vi "MotorControl.vi"() -> ()   [LabVIEW 2022 SP3]
uses:
  <vilib>/Instr/_visa.llb/VISA Configure Serial Port (Instr).vi
panel:
  in  "clear":bool
  in  "Stop":bool
  out "Console":string
  in  "Cmds":enum32{"COM Port", "Run", "Advanced"}(tab)
  in  "Test":bool
  in  "VISA resource name":refnum<visa-resource-name>
  in  "Move":bool
  in  "desired steps":i16
  in  "Angle":i16(slide) scale=0.0..360.0
  in  "on":bool
  in  "off":bool
  in  "zero":bool
  in  "read":bool
  out "angle (deg)":i16
  in  "hit":bool
  in  "steps per degree":dbl=1.67
  in  "CntrlD":bool
  in  "Play Button":bool
  in  "String":string="turn(sm,100, True)\r\n"
  in  "Download":bool
  in  "CntrlC":bool
  # "sm.irq(flip)\nsm.active(1)\nturn(sm,100, True) # one Motor rotation CCW is 200 steps\nwhile running:\n    sleep(0.5)\n\nturn(sm,100, False)\nwhile running:\n    sleep(0.5)\n\nprint(\"done\")\nsm.active(0)\nsm.exec(\"set(pins,0)\")"
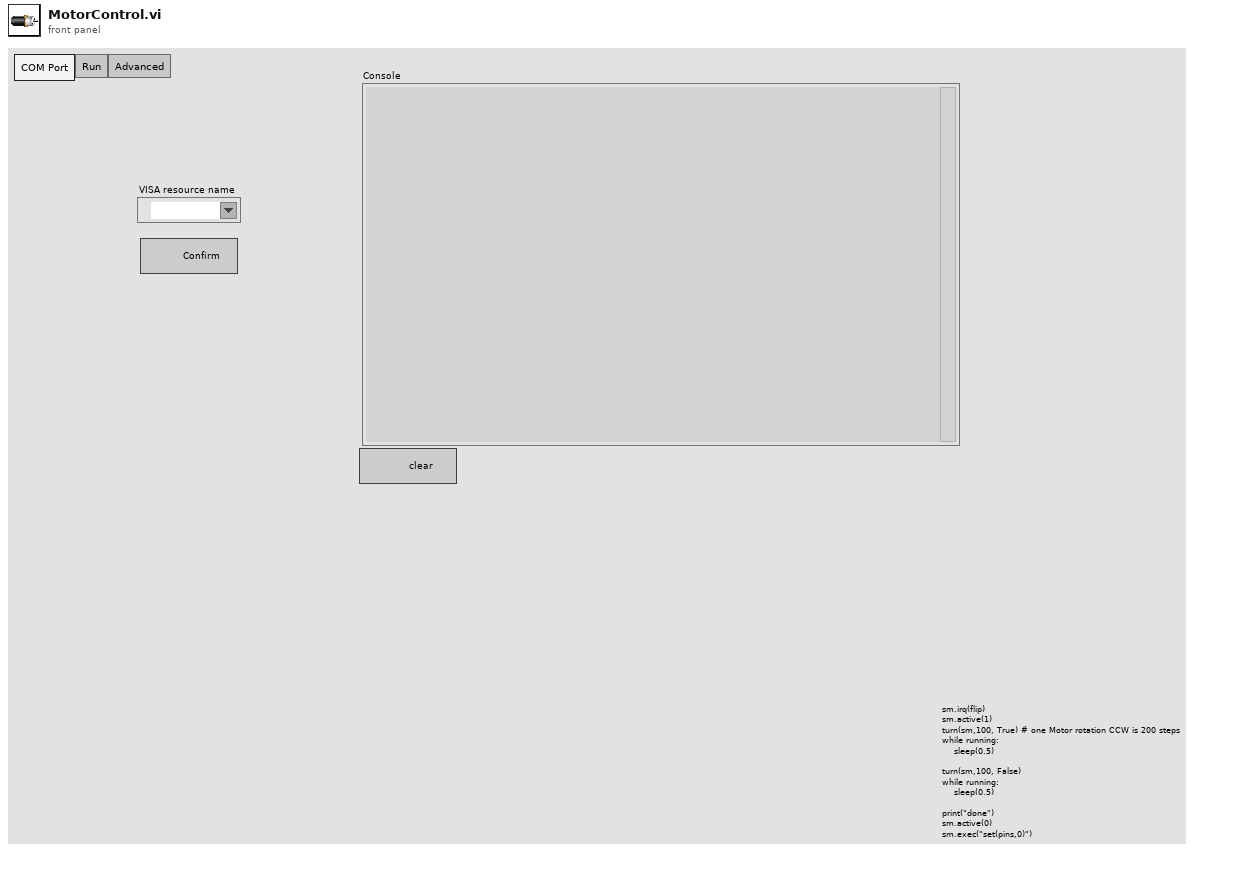
[diagram p1: front panel]
types:
  T1 = enum8{"Enabled", "Disabled", "Disabled and Grayed Out"}
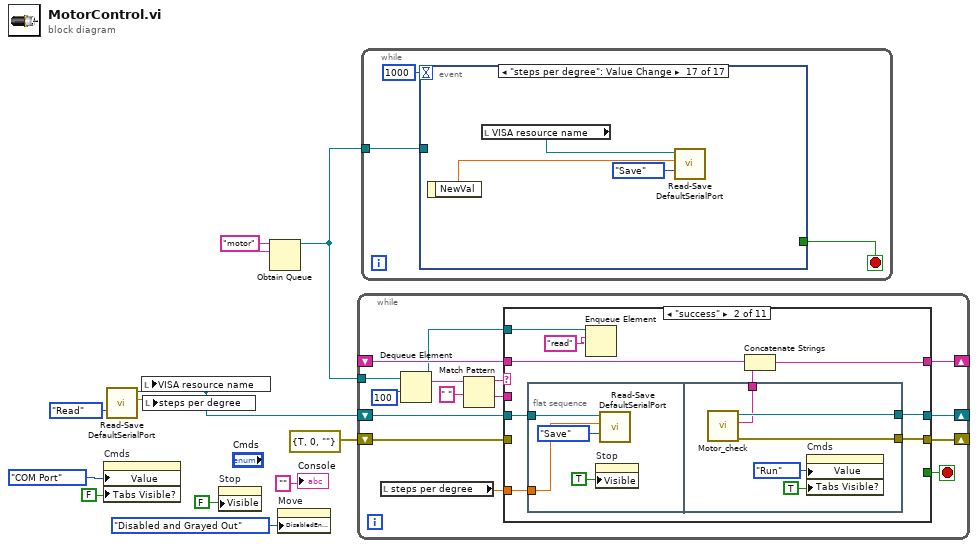
[diagram p0: block diagram]
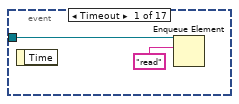
[diagram p2: hidden frame]
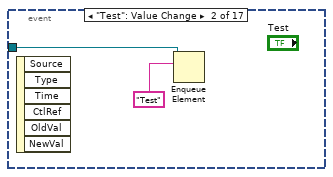
[diagram p3: hidden frame]
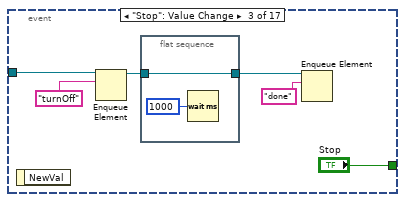
[diagram p4: hidden frame]
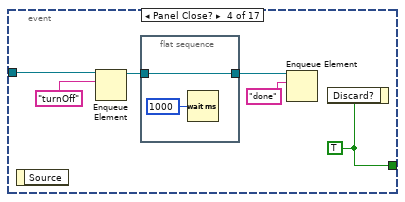
[diagram p5: hidden frame]
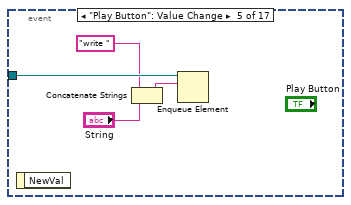
[diagram p6: hidden frame]
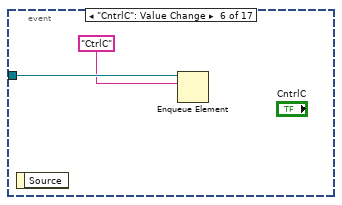
[diagram p7: hidden frame]
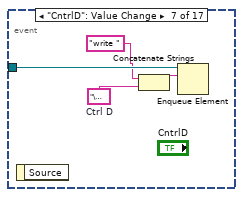
[diagram p8: hidden frame]
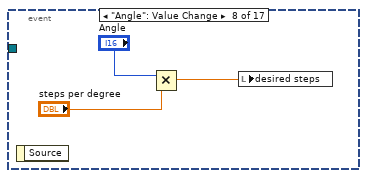
[diagram p9: hidden frame]
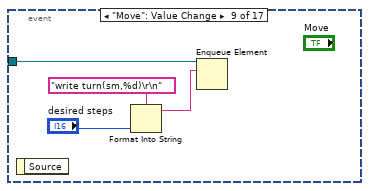
[diagram p10: hidden frame]
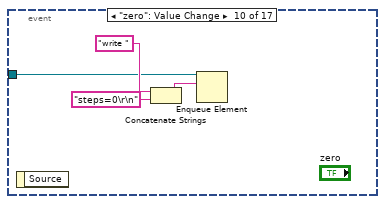
[diagram p11: hidden frame]
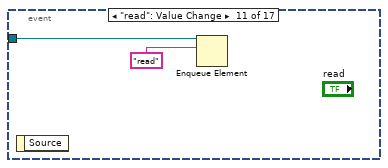
[diagram p12: hidden frame]
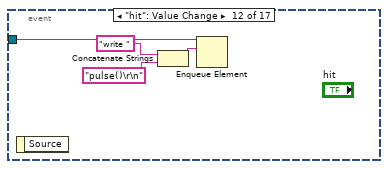
[diagram p13: hidden frame]
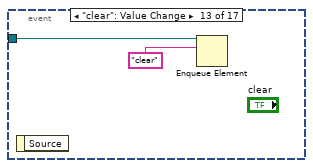
[diagram p14: hidden frame]
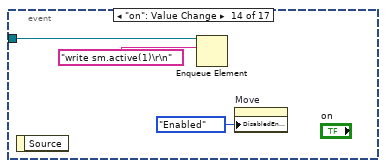
[diagram p15: hidden frame]
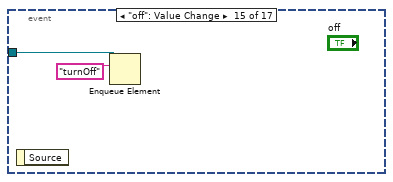
[diagram p16: hidden frame]
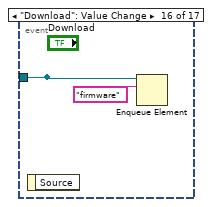
[diagram p17: hidden frame]
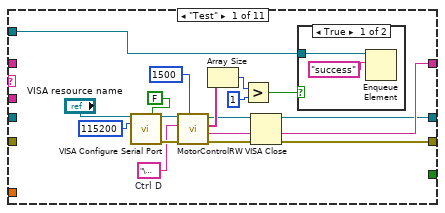
[diagram p18: hidden frame]
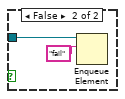
[diagram p19: hidden frame]
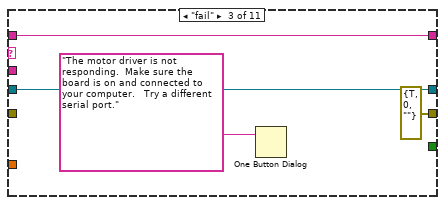
[diagram p20: hidden frame]
diagram:
  w5 = "motor" ("name (unnamed)")
  n1 = property on="Cmds" class="TabCtl (strict)"("Value"=enum32{"COM Port", "Run", "Advanced"}."COM Port" ("Cmds"), "Tabs Visible?"=FALSE) -> ()  [unwired: 2 in, 2 out]
  n2 = call "Read-Save DefaultSerialPort.vi"("Task"=enum16{"Save", "Read"}."Read") -> ("steps per degree out"=w1:dbl, "VISA out"=w4:refnum<visa-resource-name>)  [unwired: 8 in, 1 out]
  n3 = local write "VISA resource name"(w4) -> ()
  n4 = local write "steps per degree"(w1) -> ()
  n5 = property on="Stop" class="Bool"("Visible"=FALSE) -> ()  [unwired: 2 in, 2 out]
  n6 = Obtain Queue(name (unnamed)=w5, element data type=w5) -> (queue out=w3:refnum<queue>)  [unwired: 3 in, 2 out]
  n7 = property on="Move" class="Bool"("DisabledEnum"=T1."Disabled and Grayed Out" ("Disabled")) -> ()  [unwired: 2 in, 2 out]
  n8 = while {
    shift-right: [w24] -> _
    shift-left: _ -> [w25]
    tunnel: w3 -> [w22]
    shift-right: [w15] -> _
    shift-left: w4 -> [w26]
    shift-right: [w14] -> _
    shift-left: errorcluster {"status"=TRUE, "code"=0, "source"=""} ("error out") -> [w23]
    stop <- w16 stop-if-true
    n9 = local read "steps per degree"() -> (w12:dbl)
    n10 = Dequeue Element(queue=w22, timeout in ms (-1)=100) -> (queue out=w13:refnum<queue>, element=w20:string)  [unwired: 1 in, 2 out]
    n11 = Match Pattern(string=w20, regular expression=" ") -> (before substring=w19:string, after substring=w18:string)  [unwired: 1 in, 2 out]
    n12 = case shown="\"success\"" w19 {
      tunnel: w26 -> [_ w54 w66 w72 w79 w85 w94 w103 w112 w116 w127]
      tunnel: w25 -> [_ w50 w67 w68 w76 w83 w99 _ w113 w121 w126]
      tunnel: [w31 w49 w67 w69 w76 w83 w98 "" w113 w121 w125] -> w24
      tunnel: w23 -> [_ _ _ w73 w78 w84 w95 w102 w111 w117 w122]
      tunnel: w18 -> [_ _ _ _ w77 _ _ _ _ _ _]
      tunnel: [_ _ _ _ _ _ _ _ _ TRUE _] -> w16
      tunnel: [w28 w52 w66 w72 w75 w80 w97 w103 w106 w116 w124] -> w15
      tunnel: [w27 w53 errorcluster {"status"=TRUE, "code"=0, "source"=""} ("error out") w71 w74 w81 w96 w102 w105 w115 w123] -> w14
      tunnel: w13 -> [w29 w47 _ _ _ _ _ _ _ _ _]
      tunnel: w12 -> [_ w46 _ _ _ _ w86 _ _ _ _]
      frame "Test" {
        w34 = "\u0004"  # Ctrl D
        n13 = call-poly "VISA Configure Serial Port"("VISA resource name"="VISA resource name", "Enable Termination\nChar (T)"=FALSE ("Enable Termination\nChar (T)"), "baud rate (9600)"=u32 115200) -> ("VISA resource name out"=w38:refnum<visa-resource-name>, "error out"=w39:errorcluster)  [unwired: 11 in]
        n14 = call "MotorControlRW.vi"("timeout (msec)"=u32 1500 ("timeout"), "error in (no error)"=w39, "payload"=w34, "VISA in"=w38) -> ("error out"=w27:errorcluster, "reply"=w31:string, "rows"=w40:string[], "VISA Out"=w28:refnum<visa-resource-name>)  [unwired: 3 in, 1 out]
        n15 = Array Size(array=w40) -> (size(s)=w41:i32)
        n16 = Greater?(x=w41, y=1) -> (0:w30:bool)
        n17 = VISA Close(VISA resource name=w28, error in (no error)=w27) -> ()  [unwired: 1 out]
        n18 = case shown="True" w30 {
          tunnel: w29 -> [w42 w44]
          frame True {
            n19 = Enqueue Element(queue=w42, element="success") -> ()  [unwired: 2 in, 3 out]
          }
          frame False {
            n20 = Enqueue Element(queue=w44, element="fail") -> ()  [unwired: 2 in, 3 out]
          }
        }
      }
      frame "success" {
        n21 = flat-sequence {
          tunnel: w54 -> [w56]
          tunnel: w46 -> [w55]
          tunnel: [w63] -> w53
          tunnel: [w62] -> w52
          tunnel: [w59] -> w51
          frame #0 {
            n22 = property on="Stop" class="Bool"("Visible"=TRUE) -> ()  [unwired: 2 in, 2 out]
            n23 = call "Read-Save DefaultSerialPort.vi"("Task"=enum16{"Save", "Read"}."Save", "steps per degree"=w55, "VISA"=w56) -> ()  [unwired: 6 in, 3 out]
          }
          frame #1 {
            n24 = call "Motor_check.vi"() -> ("error out"=w63:errorcluster, "reply"=w59:string, "VISA Refnum out"=w62:refnum<visa-resource-name>)  [unwired: 8 in, 1 out]
            n25 = property on="Cmds" class="TabCtl (strict)"("Value"=enum32{"COM Port", "Run", "Advanced"}."Run" ("Cmds"), "Tabs Visible?"=TRUE) -> ()  [unwired: 2 in, 2 out]
          }
        }
        n26 = Enqueue Element(queue=w47, element="read") -> ()  [unwired: 2 in, 3 out]
        n27 = Concatenate Strings(w50, w51) -> (w49:string)
      }
      frame "fail" {
        n28 = One Button Dialog(message="The motor driver is not responding.  Make sure the board is on and connected to your computer.   Try a different serial port." ("regular expression")) -> ()  [unwired: 1 in, 1 out]
      }
      frame "firmware" {
        n29 = call "Motor_firmware.vi"("error in (no error)"=w73, "VISA Refnum in"=w72) -> ("error out"=w71:errorcluster, "reply"=w70:string)  [unwired: 8 in]
        n30 = Concatenate Strings(w68, w70) -> (w69:string)
      }
      frame "write" {
        n31 = VISA Write(VISA resource name=w79, write buffer=w77, error in (no error)=w78) -> (VISA resource name out=w75:refnum<visa-resource-name>, error out=w74:errorcluster)  [unwired: 1 out]
      }
      frame "CtrlC" {
        w82 = "\u0003"  # Ctrl C
        n32 = VISA Write(VISA resource name=w85, write buffer=w82, error in (no error)=w84) -> (VISA resource name out=w80:refnum<visa-resource-name>, error out=w81:errorcluster)  [unwired: 1 out]
      }
      frame "read" {
        w100 = "steps\r\n"  # steps?
        n33 = call "MotorControlRW.vi"("error in (no error)"=w95, "payload"=w100, "VISA in"=w94) -> ("error out"=w96:errorcluster, "reply"=w92:string, "rows"=w101:string[], "VISA Out"=w97:refnum<visa-resource-name>)  [unwired: 4 in, 1 out]
        n34 = Index Array(array=w101) -> (element #2=w90:string)  [unwired: 2 in, 1 out]
        n35 = Decimal String To Number(string=w90) -> (number=w89:i32)  [unwired: 2 in, 1 out]
        n36 = Match Pattern(string=w92, regular expression="steps") -> (before substring=w91:string)  [unwired: 1 in, 3 out]
        n37 = Divide(x=w89, y=w86) -> (x/y=w88:dbl)
        n38 = Round To Nearest(number=w88) -> (nearest integer value=→"angle (deg)":dbl)
        n39 = Concatenate Strings(w99, w91) -> (w98:string)
      }
      frame "clear" {
      }
      frame "turnOff" {
        w110 = "\u0003"  # Ctrl C
        n40 = VISA Write(VISA resource name=w112, write buffer=w110, error in (no error)=w111) -> (VISA resource name out=w109:refnum<visa-resource-name>, error out=w108:errorcluster)  [unwired: 1 out]
        n41 = VISA Write(VISA resource name=w109, write buffer="sm.active(0)\r\nsm.exec(\"set(pins,0)\")\r\n" ("element"), error in (no error)=w108) -> (VISA resource name out=w106:refnum<visa-resource-name>, error out=w105:errorcluster)  [unwired: 1 out]
        n42 = property on="Move" class="Bool"("DisabledEnum"=T1."Disabled and Grayed Out" ("Disabled")) -> ()  [unwired: 2 in, 2 out]
      }
      frame "done" {
        n43 = VISA Close(VISA resource name=w116, error in (no error)=w117) -> (error out=w115:errorcluster)
        n44 = property on="Cmds" class="TabCtl (strict)"("Value"=enum32{"COM Port", "Run", "Advanced"}."COM Port" ("Cmds"), "Tabs Visible?"=TRUE) -> ()  [unwired: 2 in, 2 out]
      }
      frame Default {
        n45 = case shown="No Error" w122 {
          selector: w122 -> [w128 w139]
          tunnel: w127 -> [w135 w140]
          tunnel: w126 -> [w133 w141]
          tunnel: [w132 w141] -> w125
          tunnel: [w130 w140] -> w124
          tunnel: [w129 w139] -> w123
          frame No Error {
            n46 = property class="Instr"(reference=w135, error in=w128) -> (reference out=w138:refnum<visa-resource-name>, error out=w136:errorcluster, "Serial Settings:Number of Bytes at Serial Port"=w137:u32)
            n47 = VISA Read(VISA resource name=w138, byte count=w137, error in (no error)=w136) -> (VISA resource name out=w130:refnum<visa-resource-name>, read buffer=w134:string, error out=w129:errorcluster)  [unwired: 1 out]
            n48 = Concatenate Strings(w133, w134) -> (w132:string)
            n49 = property on="Console" class="Str"("Value"=w132, "Text.Scroll Position"=u32 999999) -> ()  [unwired: 2 in, 2 out]
          }
          frame Error {
          }
        }
      }
    }
  }
  n50 = while {
    tunnel: w3 -> [w144]
    stop <- w143 stop-if-true
    n51 = event shown="[16] \"steps per degree\": Value Change" {
      selector: _ -> [_ _ _ _ _ _ _ _ _ _ _ _ _ _ _ _ _]
      dyn-events: _ -> [_ _ _ _ _ _ _ _ _ _ _ _ _ _ _ _ _]
      timeout: 1000 -> [_ _ _ _ _ _ _ _ _ _ _ _ _ _ _ _ _]
      tunnel: w144 -> [w146 w148 w152 w161 w168 w170 w174 _ w181 w183 w187 w191 w193 w196 w198 w200 _]
      tunnel: [_ _ "Stop" w157 _ _ _ _ _ _ _ _ _ _ _ _ _] -> w143
      tunnel: [_ _ _ _ _ _ _ _ _ _ _ _ _ _ _ w200 _] -> _
      event Timeout {
        n52 = event-data() -> ()  [unwired: 1 in, 1 out]
        n53 = Enqueue Element(queue=w146, element="read") -> ()  [unwired: 2 in, 3 out]
      }
      event "Test": Value Change {
        n54 = event-data() -> ()  [unwired: 1 in, 6 out]
        n55 = Enqueue Element(queue=w148, element="Test") -> ()  [unwired: 2 in, 3 out]
      }
      event "Stop": Value Change {
        n56 = event-data() -> ()  [unwired: 1 in, 1 out]
        n57 = Enqueue Element(queue=w152, element="turnOff") -> (queue out=w149:refnum<queue>)  [unwired: 2 in, 2 out]
        n58 = flat-sequence {
          tunnel: [w156] -> w150
          tunnel: w149 -> [w156]
          frame #0 {
            n59 = Wait (ms)(milliseconds to wait=u32 1000) -> ()  [unwired: 1 out]
          }
        }
        n60 = Enqueue Element(queue=w150, element="done") -> ()  [unwired: 2 in, 3 out]
      }
      event Panel Close? {
        w157 = TRUE
        n61 = event-data() -> ()  [unwired: 1 in, 1 out]
        n62 = Enqueue Element(queue=w161, element="turnOff") -> (queue out=w158:refnum<queue>)  [unwired: 2 in, 2 out]
        n63 = flat-sequence {
          tunnel: [w164] -> w159
          tunnel: w158 -> [w164]
          frame #0 {
            n64 = Wait (ms)(milliseconds to wait=u32 1000) -> ()  [unwired: 1 out]
          }
        }
        n65 = Enqueue Element(queue=w159, element="done") -> ()  [unwired: 2 in, 3 out]
        n66 = event-data("Discard?"=w157) -> ()  [unwired: 1 in, 1 out]
      }
      event "Play Button": Value Change {
        n67 = event-data() -> ()  [unwired: 1 in, 1 out]
        n68 = Concatenate Strings("write " ("element"), "String") -> (w165:string)
        n69 = Enqueue Element(queue=w168, element=w165) -> ()  [unwired: 2 in, 3 out]
      }
      event "CntrlC": Value Change {
        n70 = event-data() -> ()  [unwired: 1 in, 1 out]
        n71 = Enqueue Element(queue=w170, element="CtrlC") -> ()  [unwired: 2 in, 3 out]
      }
      event "CntrlD": Value Change {
        w172 = "\u0004"  # Ctrl D
        n72 = event-data() -> ()  [unwired: 1 in, 1 out]
        n73 = Concatenate Strings("write " ("element"), w172) -> (w171:string)
        n74 = Enqueue Element(queue=w174, element=w171) -> ()  [unwired: 2 in, 3 out]
      }
      event "Angle": Value Change {
        n75 = event-data() -> ()  [unwired: 1 in, 1 out]
        n76 = Multiply(x="Angle", y="steps per degree") -> (x*y=w175:dbl)
        n77 = local write "desired steps"(w175) -> ()
      }
      event "Move": Value Change {
        n78 = event-data() -> ()  [unwired: 1 in, 1 out]
        n79 = Format Into String(format string="write turn(sm,%d)\r\n" ("string"), "desired steps") -> (resulting string=w178:string)  [unwired: 2 in, 1 out]
        n80 = Enqueue Element(queue=w181, element=w178) -> ()  [unwired: 2 in, 3 out]
      }
      event "zero": Value Change {
        n81 = event-data() -> ()  [unwired: 1 in, 1 out]
        n82 = Concatenate Strings("write " ("element"), "steps=0\r\n" ("string")) -> (w185:string)
        n83 = Enqueue Element(queue=w183, element=w185) -> ()  [unwired: 2 in, 3 out]
      }
      event "read": Value Change {
        n84 = event-data() -> ()  [unwired: 1 in, 1 out]
        n85 = Enqueue Element(queue=w187, element="read") -> ()  [unwired: 2 in, 3 out]
      }
      event "hit": Value Change {
        n86 = event-data() -> ()  [unwired: 1 in, 1 out]
        n87 = Concatenate Strings("write " ("element"), "pulse()\r\n" ("string")) -> (w188:string)
        n88 = Enqueue Element(queue=w191, element=w188) -> ()  [unwired: 2 in, 3 out]
      }
      event "clear": Value Change {
        n89 = event-data() -> ()  [unwired: 1 in, 1 out]
        n90 = Enqueue Element(queue=w193, element="clear") -> ()  [unwired: 2 in, 3 out]
      }
      event "on": Value Change {
        n91 = event-data() -> ()  [unwired: 1 in, 1 out]
        n92 = Enqueue Element(queue=w196, element="write sm.active(1)\r\n" ("string")) -> ()  [unwired: 2 in, 3 out]
        n93 = property on="Move" class="Bool"("DisabledEnum"=T1."Enabled" ("Disabled")) -> ()  [unwired: 2 in, 2 out]
      }
      event "off": Value Change {
        n94 = event-data() -> ()  [unwired: 1 in, 1 out]
        n95 = Enqueue Element(queue=w198, element="turnOff") -> ()  [unwired: 2 in, 3 out]
      }
      event "Download": Value Change {
        n96 = event-data() -> ()  [unwired: 1 in, 1 out]
        n97 = Enqueue Element(queue=w200, element="firmware") -> ()  [unwired: 2 in, 3 out]
      }
      event "steps per degree": Value Change {
        n98 = event-data() -> ("NewVal"=w202:dbl)  [unwired: 1 in]
        n99 = local read "VISA resource name"() -> (w201:refnum<visa-resource-name>)
        n100 = call "Read-Save DefaultSerialPort.vi"("Task"=enum16{"Save", "Read"}."Save", "steps per degree"=w202, "VISA"=w201) -> ()  [unwired: 6 in, 3 out]
      }
    }
  }
  "Console" <- "" ("element")
